vi "Startup.vi"   [LabVIEW 2015]
uses:
  <userlib>/Newport ESP301/Newport ESP301.lvlib
panel:
  # "With the ESP301 on, run this program and it will find and set the mid point of all axes to zero."
types:
  T1 = enum16{"Trapezoidal Mode", "S-curve Mode", "Jog Mode", "Slave to master's desired position (trajectory)", "Slave to master's actual position (feedback)", "Slave to master's actual velocity for jogging"}
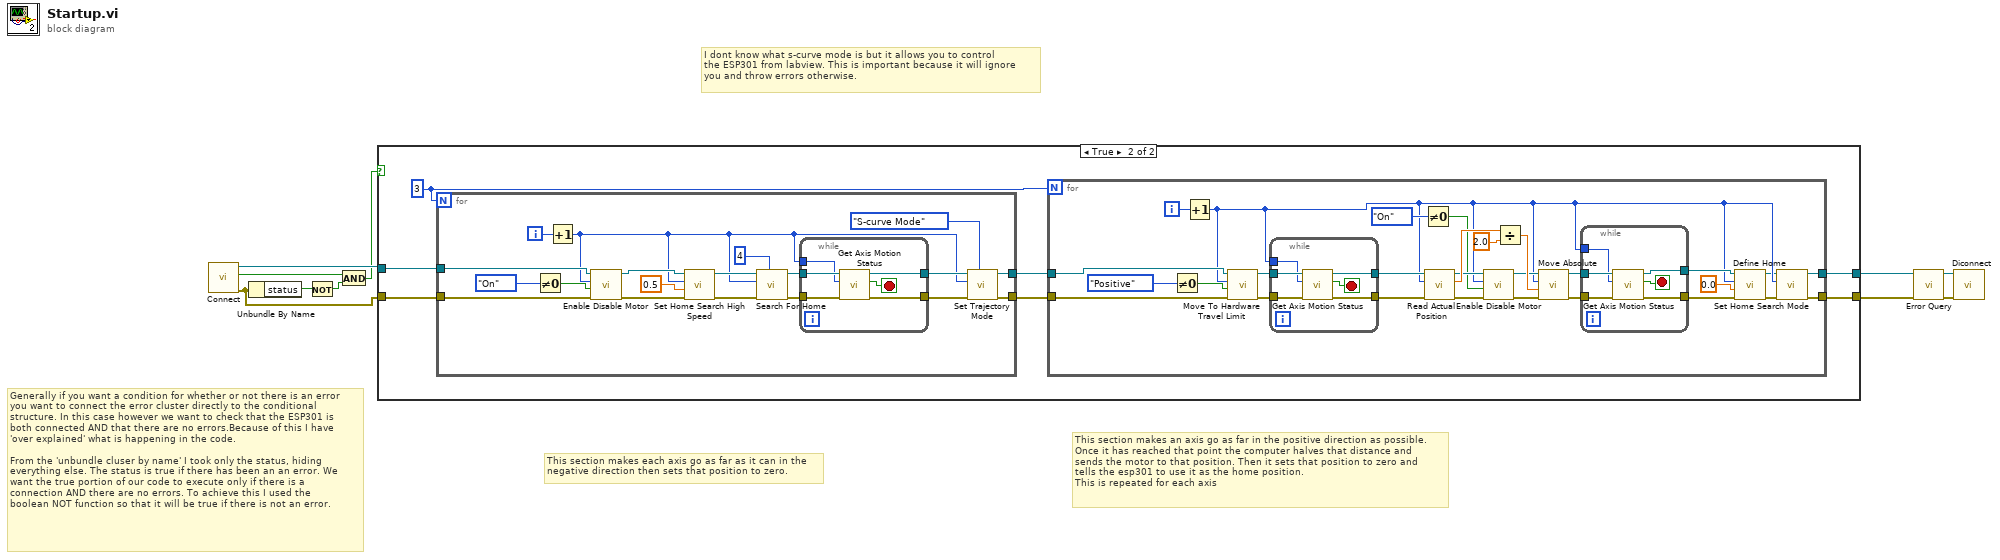
[diagram p0: block diagram]
diagram:
  # "This section makes an axis go as far in the positive direction as possible. \nOnce it has reached that point the computer halves that distance and\nsends the motor to that position. Then it sets that position to zero and \ntells the esp301 to use it as the home position. \nThis is repeated for each axis"
  # "This section makes each axis go as far as it can in the \nnegative direction then sets that position to zero."
  # "I dont know what s-curve mode is but it allows you to control \nthe ESP301 from labview. This is important because it will ignore \nyou and throw errors otherwise."
  # "Generally if you want a condition for whether or not there is an error\nyou want to connect the error cluster directly to the conditional\nstructure. In this case however we want to check that the ESP301 is\nboth connected AND that there are no errors.Because of this I have\n'over explained' what is happening in the code.\n\nFrom the 'unbundle cluser by name' I took only the status, hiding \neverything else. The status is true if there has been an an error. We\nwant the true portion of our code to execute only if there is a \nconnection AND there are no errors. To achieve this I used the \nboolean NOT function so that it will be true if there is not an error."
  n1 = call "Connect.vi"() -> ("error out"=w9:errorcluster, "Connected"=w1:bool, "VISA resource name out"=w10:refnum<visa-resource-name>)  [unwired: 5 in]
  n2 = Unbundle By Name(w9) -> ("status"=w8:bool)
  n3 = Not(x=w8) -> (.not. x?=w2:bool)
  n4 = And(x=w1, y=w2) -> (x .and. y?=w3:bool)
  n5 = case shown="True" w3 {
    tunnel: w10 -> [w12 w19]
    tunnel: w9 -> [w11 w18]
    tunnel: [w12 w14] -> w7
    tunnel: [w11 w13] -> w6
    frame False {
    }
    frame True {
      w17 = 3
      n6 = for {
        N: w17 -> [_]
        tunnel: w19 -> [w66]
        tunnel: w18 -> [w65]
        tunnel: [w73] -> w16
        tunnel: [w72] -> w15
        i -> [w78]
        n7 = Not Equal To 0?(x=enum16{"Off", "On"}."On") -> (x != 0?=w60:bool)
        n8 = Increment(x=w78) -> (x+1=w62:i32)
        n9 = call <userlib>:"Enable Disable Motor.vi"("error in (no error)"=w65, "Action (F - OFF)"=w60, "Axis (1)"=w62, "VISA resource name"=w66) -> ("error out"=w63:errorcluster, "VISA resource name out"=w64:refnum<visa-resource-name>)  [unwired: 2 in]
        n10 = call <userlib>:"Set Home Search High Speed.vi"("error in (no error)"=w63, "Search High Speed (0 units/s)"=0.5, "Axis (1)"=w62, "VISA resource name"=w64) -> ("error out"=w76:errorcluster, "VISA resource name out"=w77:refnum<visa-resource-name>)  [unwired: 2 in]
        n11 = call <userlib>:"Search For Home.vi"("Home mode"=4, "error in (no error)"=w76, "Axis (1)"=w62, "VISA resource name"=w77) -> ("error out"=w69:errorcluster, "VISA resource name out"=w70:refnum<visa-resource-name>)  [unwired: 3 in]
        n12 = while {
          tunnel: w70 -> [w84]
          tunnel: w69 -> [w83]
          tunnel: w62 -> [w82]
          tunnel: [w81] -> w68
          tunnel: [w80] -> w67
          stop <- w79 stop-if-true
          n13 = call <userlib>:"Get Axis Motion Status.vi"("error in (no error)"=w83, "Axis (1)"=w82, "VISA resource name"=w84) -> ("error out"=w80:errorcluster, "Motion Done"=w79:bool, "VISA resource name out"=w81:refnum<visa-resource-name>)  [unwired: 2 in]
        }
        n14 = call <userlib>:"Set Trajectory Mode.vi"("Trajectory Mode"=T1."S-curve Mode", "error in (no error)"=w67, "Axis (1)"=w62, "VISA resource name"=w68) -> ("error out"=w72:errorcluster, "VISA resource name out"=w73:refnum<visa-resource-name>)  [unwired: 3 in]
      }
      n15 = for {
        N: w17 -> [_]
        tunnel: w16 -> [w46]
        tunnel: w15 -> [w45]
        tunnel: [w21] -> w14
        tunnel: [w20] -> w13
        i -> [w47]
        n16 = Not Equal To 0?(x=enum16{"Negative", "Positive"}."Positive") -> (x != 0?=w25:bool)
        n17 = Increment(x=w47) -> (x+1=w24:i32)
        n18 = call <userlib>:"Move To Hardware Travel Limit.vi"("error in (no error)"=w45, "Move Direction (+)"=w25, "Axis (1)"=w24, "VISA resource name"=w46) -> ("error out"=w43:errorcluster, "VISA resource name out"=w44:refnum<visa-resource-name>)  [unwired: 2 in]
        n19 = while {
          tunnel: w44 -> [w59]
          tunnel: w43 -> [w58]
          tunnel: w24 -> [w57]
          tunnel: [w56] -> w42
          tunnel: [w55] -> w41
          stop <- w54 stop-if-true
          n20 = call <userlib>:"Get Axis Motion Status.vi"("error in (no error)"=w58, "Axis (1)"=w57, "VISA resource name"=w59) -> ("error out"=w55:errorcluster, "Motion Done"=w54:bool, "VISA resource name out"=w56:refnum<visa-resource-name>)  [unwired: 2 in]
        }
        n21 = Not Equal To 0?(x=enum16{"Off", "On"}."On") -> (x != 0?=w27:bool)
        n22 = call <userlib>:"Read Actual Position.vi"("error in (no error)"=w41, "Axis (1)"=w24, "VISA resource name"=w42) -> ("error out"=w34:errorcluster, "Position (units)"=w40:dbl, "VISA resource name out"=w35:refnum<visa-resource-name>)  [unwired: 2 in]
        n23 = call <userlib>:"Enable Disable Motor.vi"("error in (no error)"=w34, "Action (F - OFF)"=w27, "Axis (1)"=w24, "VISA resource name"=w35) -> ("error out"=w33:errorcluster, "VISA resource name out"=w32:refnum<visa-resource-name>)  [unwired: 2 in]
        n24 = Divide(x=w40, y=2.0) -> (x/y=w38:dbl)
        n25 = call <userlib>:"Move Absolute.vi"("error in (no error)"=w33, "Position (0 units)"=w38, "Axis (1)"=w24, "VISA resource name"=w32) -> ("error out"=w36:errorcluster, "VISA resource name out"=w37:refnum<visa-resource-name>)  [unwired: 2 in]
        n26 = while {
          tunnel: w37 -> [w53]
          tunnel: w36 -> [w52]
          tunnel: w24 -> [w51]
          tunnel: [w50] -> w31
          tunnel: [w49] -> w30
          stop <- w48 stop-if-true
          n27 = call <userlib>:"Get Axis Motion Status.vi"("error in (no error)"=w52, "Axis (1)"=w51, "VISA resource name"=w53) -> ("error out"=w49:errorcluster, "Motion Done"=w48:bool, "VISA resource name out"=w50:refnum<visa-resource-name>)  [unwired: 2 in]
        }
        n28 = call <userlib>:"Define Home.vi"("error in (no error)"=w30, "Home Position (0 units)"=0.0, "Axis (1)"=w24, "VISA resource name"=w31) -> ("error out"=w22:errorcluster, "VISA resource name out"=w23:refnum<visa-resource-name>)  [unwired: 2 in]
        n29 = call <userlib>:"Set Home Search Mode.vi"("error in (no error)"=w22, "Axis (1)"=w24, "VISA resource name"=w23) -> ("error out"=w20:errorcluster, "VISA resource name out"=w21:refnum<visa-resource-name>)  [unwired: 4 in]
      }
    }
  }
  n30 = call <userlib>:"Error Query.vi"("error in (no error)"=w6, "VISA resource name"=w7) -> ("error out"=w5:errorcluster, "VISA resource name out"=w4:refnum<visa-resource-name>)  [unwired: 2 in, 2 out]
  n31 = call "Diconnect.vi"("error in (no error)"=w5, "VISA resource name"=w4) -> ()  [unwired: 6 in]
